vi "fgv_DL950_visa.vi"(7 "cmd":T2, 8 "error in":errorcluster, 10 "ms":u32, 11 "Initiate":string=":STAR;") -> (0 "error out":errorcluster, 2 "items":dbl[][](array[numeric]), 3 "Data":string)   [LabVIEW 2019]
uses:
  _ctrl/fgv_DL950.ctl
  _ctrl/init-r-stop.ctl
  _ctrl/rw.ctl
  SubVIs/common/cmd_err.ctl
  Durability/DL950_wfms.ctl
  d5429c9e-11ee-4f4d-90f7-2d4e6cc73670.vi
  SubVIs/common/Glob_Ref.vi
  Durability/common/Global 1.vi
  <instrlib>/Yokogawa DL950 Series/Public/Configure/Configure Module (Voltage).vi
  <instrlib>/Yokogawa DL950 Series/Public/Configure/Configure Module (Temperature).vi
  <instrlib>/Yokogawa DL950 Series/Yokogawa DL950 Series.lvlib
panel:
  out "resulting string":string
  out "Array":T1(array[cluster])
  in  "High":dbl
  in  "Middle":dbl
  in  "low":dbl
  in  "ch":i32
  out "DL950 wfm":waveform(dbl)[](graph)
  out "wf,":waveform(dbl)[](graph)
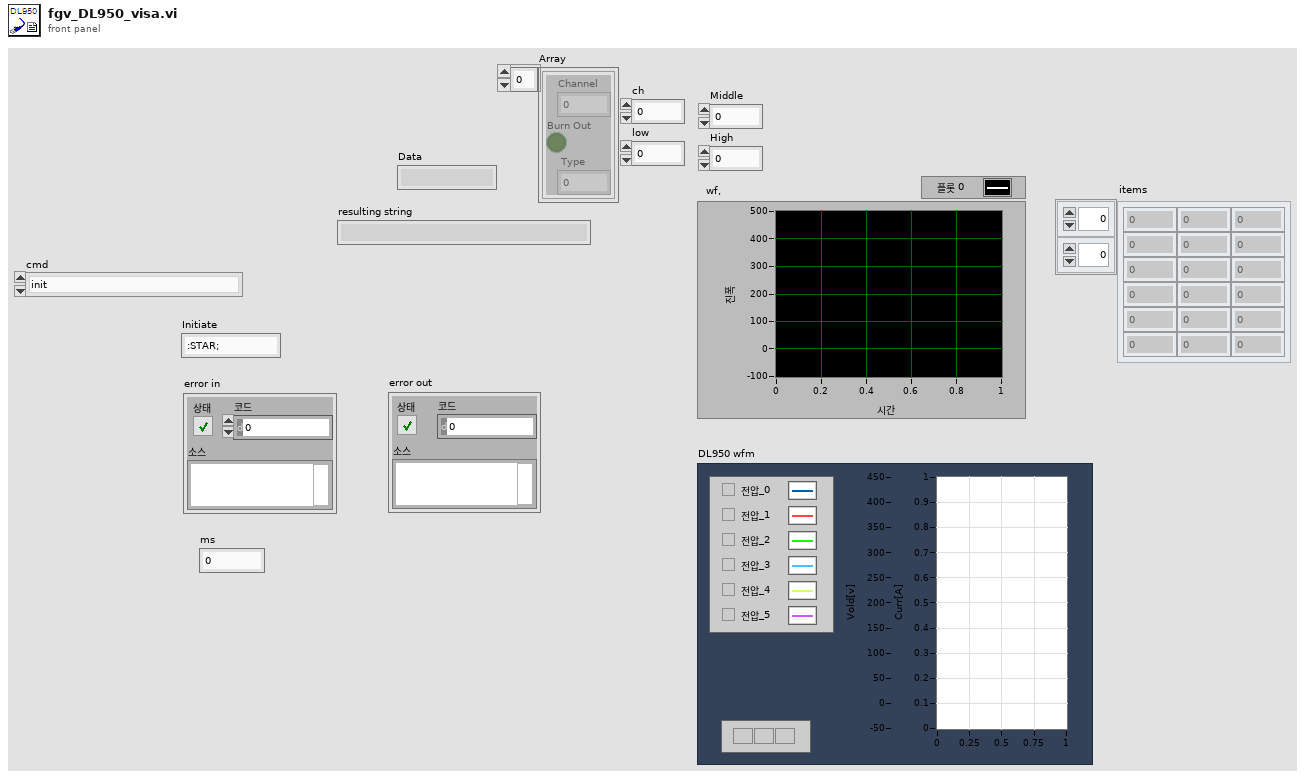
[diagram p1: front panel]
types:
  T1 = cluster{"Channel":u16, "Burn Out":bool, " Type ":i32}[]
  T2 = typedef "fgv_DL950.ctl" = enum16{"init", "config", "Set-NCh", "setapply", "trigger", "history_clear", "read", "time-div", "wave-aquis", "start", "query", "abort", "set_items", "reset_items", "read_items", "percent_rise", "trigger_single", "stop", "offset cancel", "close"}
  T3 = enum16{"DL950", "BP4610", "DSP1500", "cDAQ-AI", "cDAQ-AO", "cDAQ-DO"}
  T4 = typedef "init-r-stop.ctl" = enum16{"ini", "read", "stop"}
  T5 = typedef "cmd_err.ctl" = enum16{"close", "open", "default"}
  T6 = typedef "rw.ctl" = enum16{"read", "write"}
  T7 = typedef "DL950_wfms.ctl" = cluster{"wfms":waveform(dbl)[], "Waveform_2":cluster{"t0":dbl, "dt":dbl, "Y":dbl[][]}, "items":dbl[][], "da950_array":dbl[]}
  T8 = cluster{"Waveform_DLM5038":cluster{"l":dbl, "dt":dbl, "Y":dbl[][]}, "wf,":waveform(dbl)[]}
  T9 = typedef "DL950_config.ctl" = cluster{"Timeout":u32, "Time Div":i32, "Acq Mode":i32, "Record Len":i32, "Record Num":i32, "Start Point":i64, "End Poin":i64, "Visa":refnum<visa-resource-name>, "Config Voltage":cluster{"Enable":bool, "Ch":u16, "V Div":i32, "Coupling":i32, "Probe":i32, "Act.Items":bool, "items":i32[]}[], "Trigger on":bool, "Trigger Level":dbl, "Reset":bool, "Config Temp":cluster{"Channel":u16, "Burn Out":bool, " Type ":i32}[], "Trig Mode":i32, "Trig Pos":dbl, "Trigger Slope":i32, "Trigger Source ":i32, "Trig Start -5":dbl, "End 5":dbl}
  T10 = cluster{"Enable":bool, "Ch":u16, "V Div":i32, "Coupling":i32, "Probe":i32, "Act.Items":bool, "items":i32[]}[]
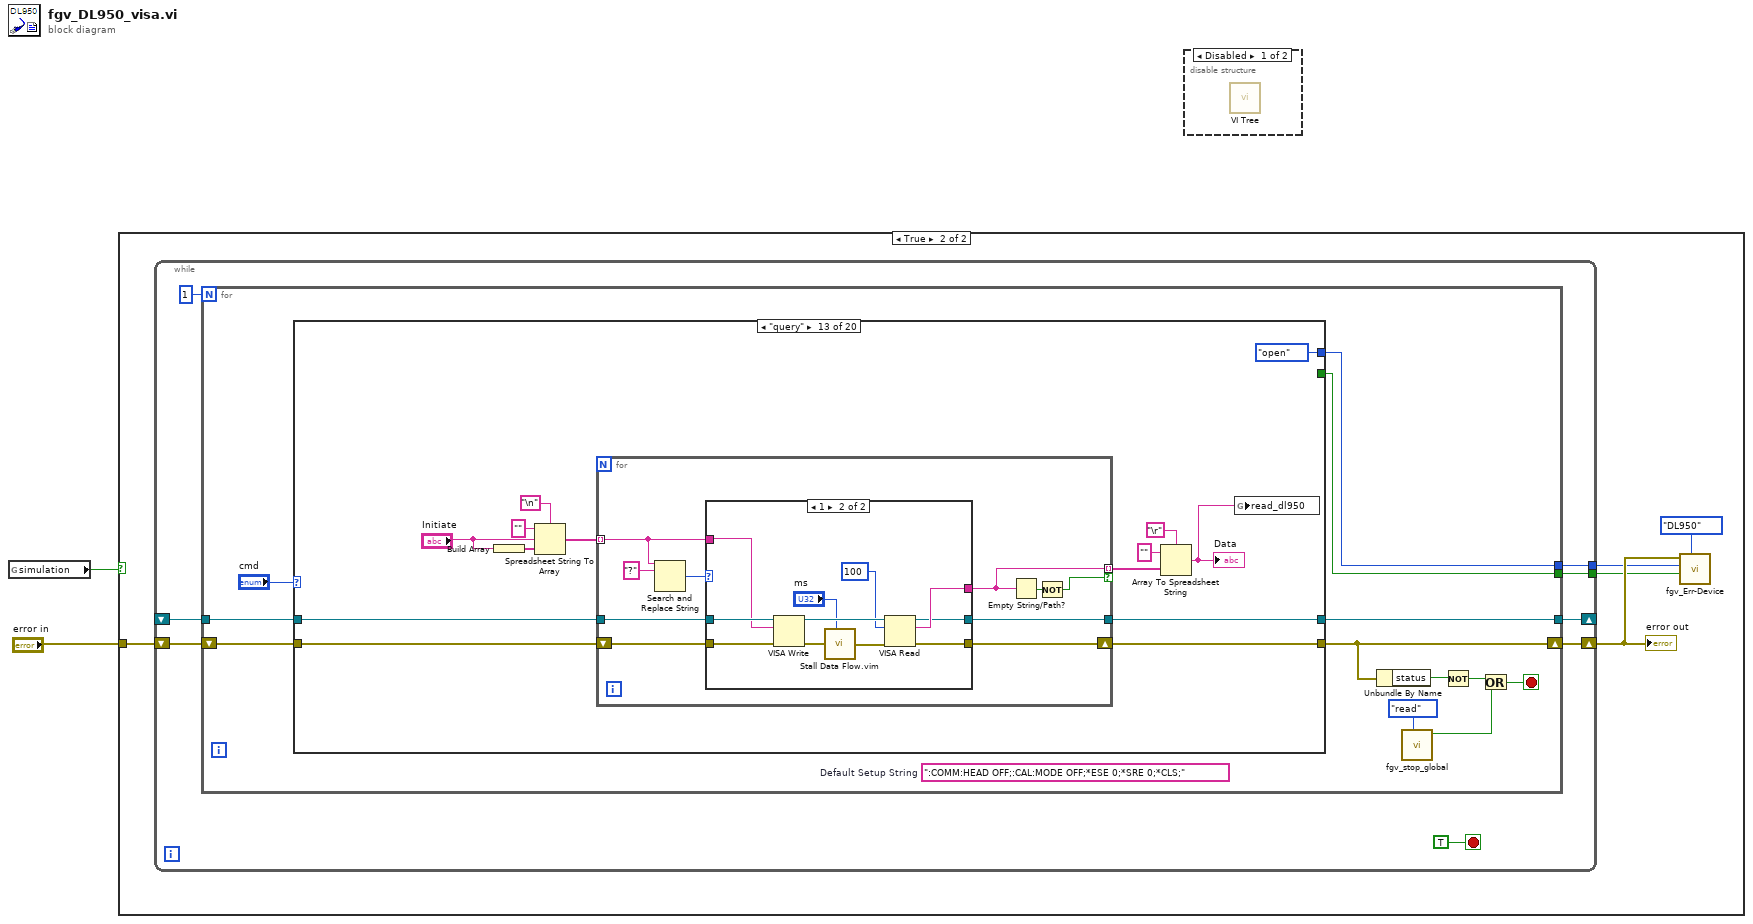
[diagram p0: block diagram]
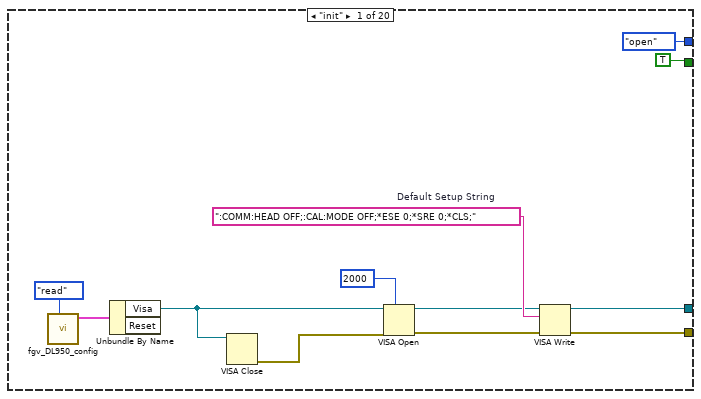
[diagram p3: hidden frame]
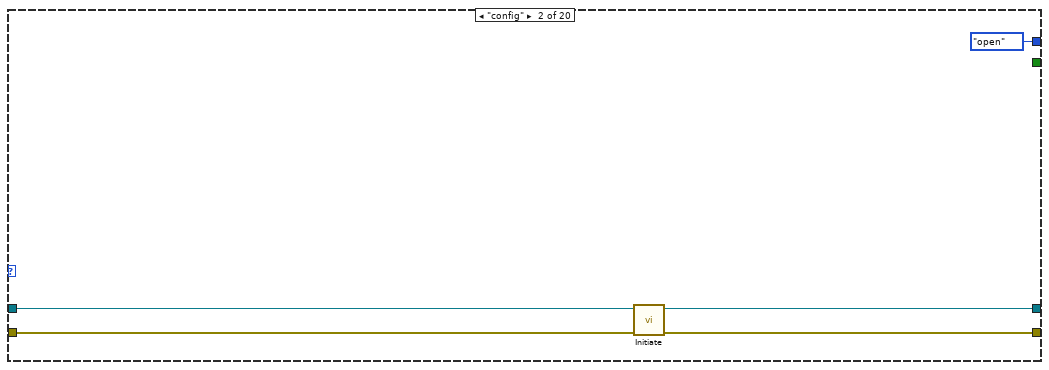
[diagram p4: hidden frame]
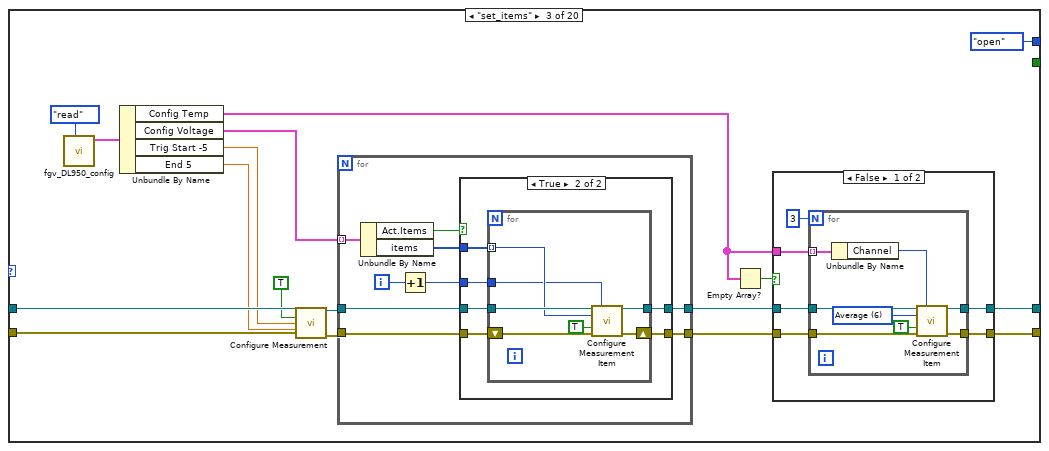
[diagram p5: hidden frame]
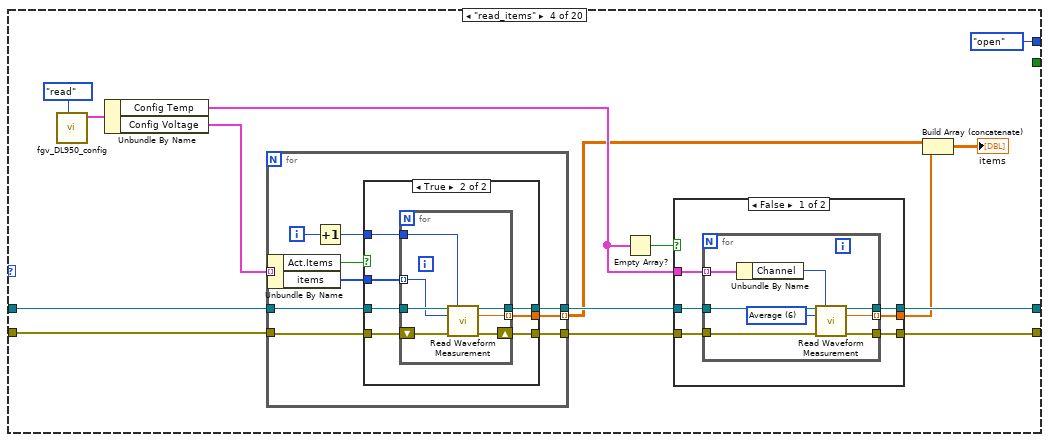
[diagram p8: hidden frame]
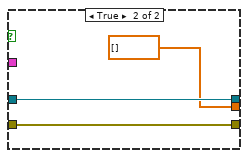
[diagram p9: hidden frame]
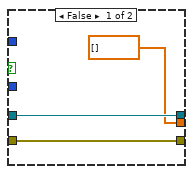
[diagram p10: hidden frame]
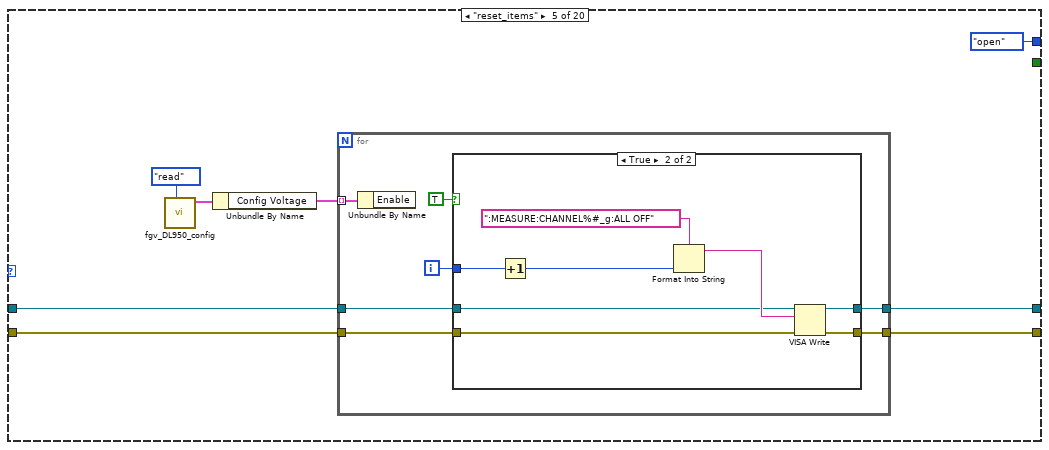
[diagram p11: hidden frame]
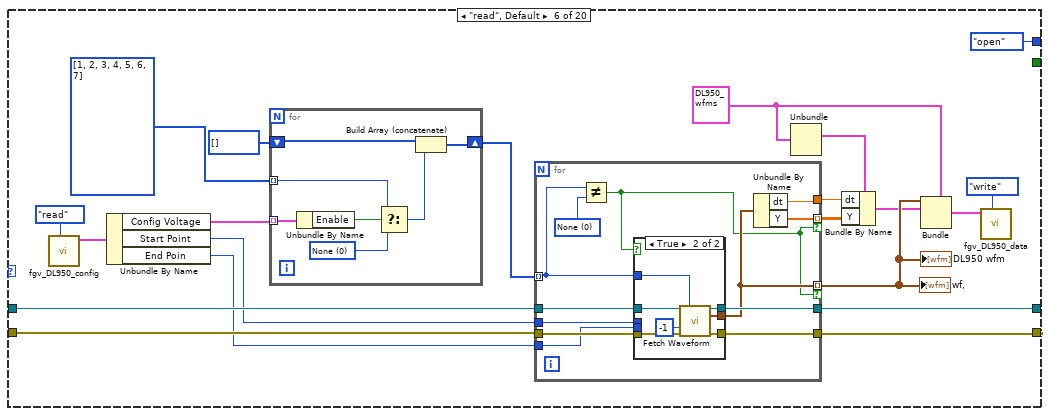
[diagram p13: hidden frame]
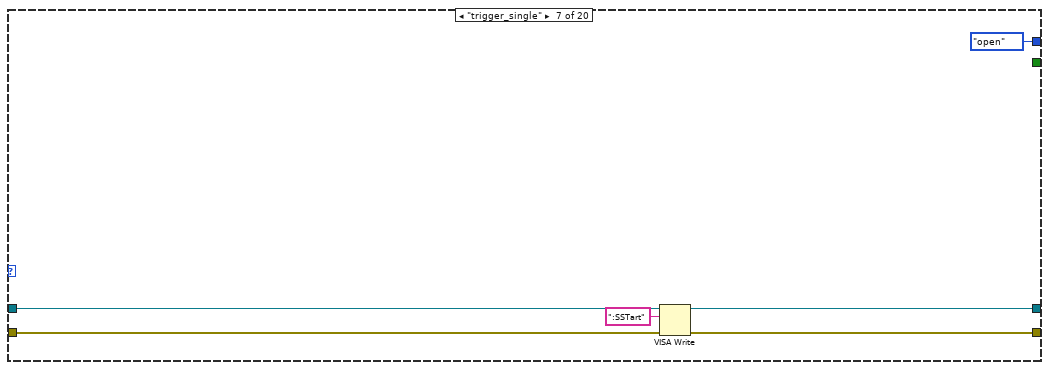
[diagram p15: hidden frame]
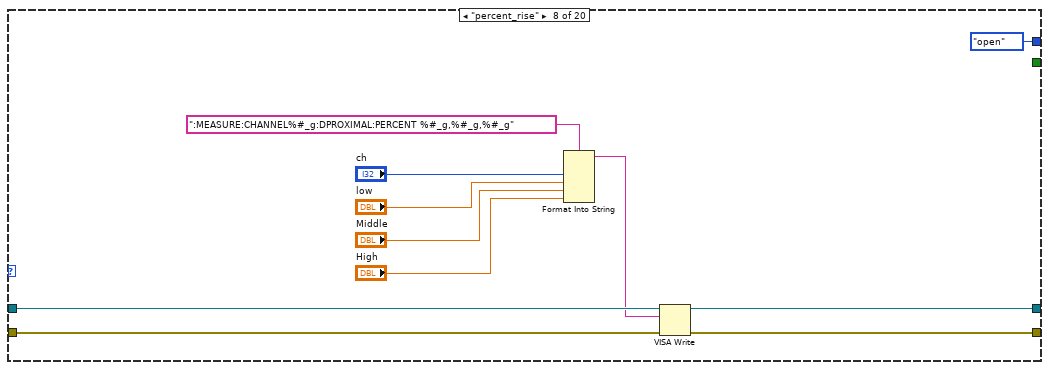
[diagram p16: hidden frame]
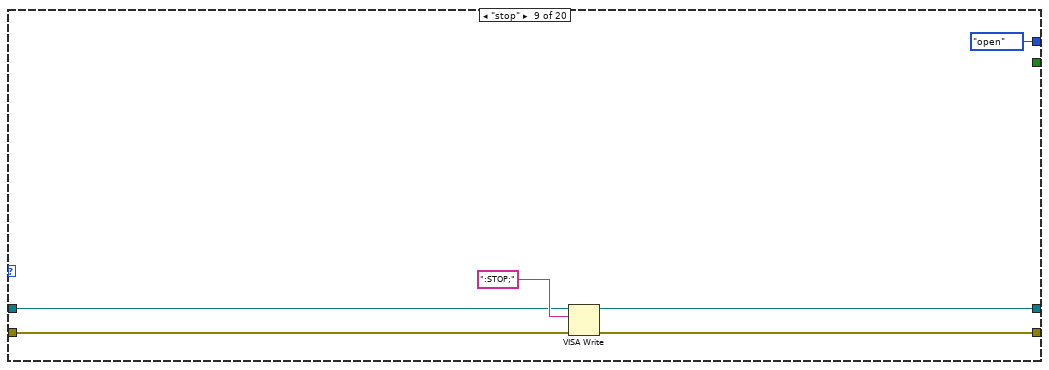
[diagram p17: hidden frame]
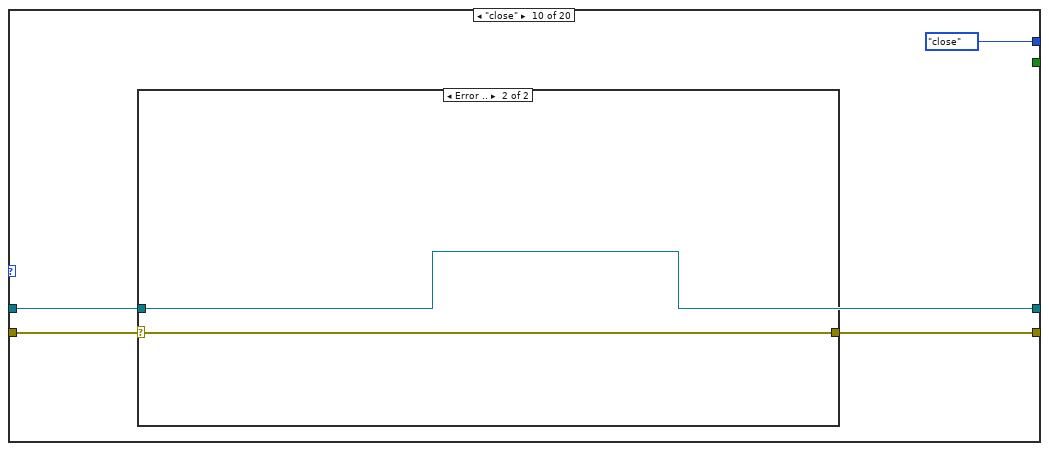
[diagram p18: hidden frame]
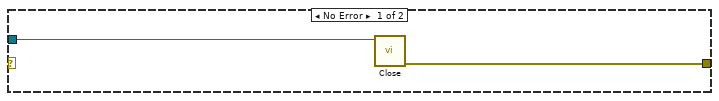
[diagram p19: hidden frame]
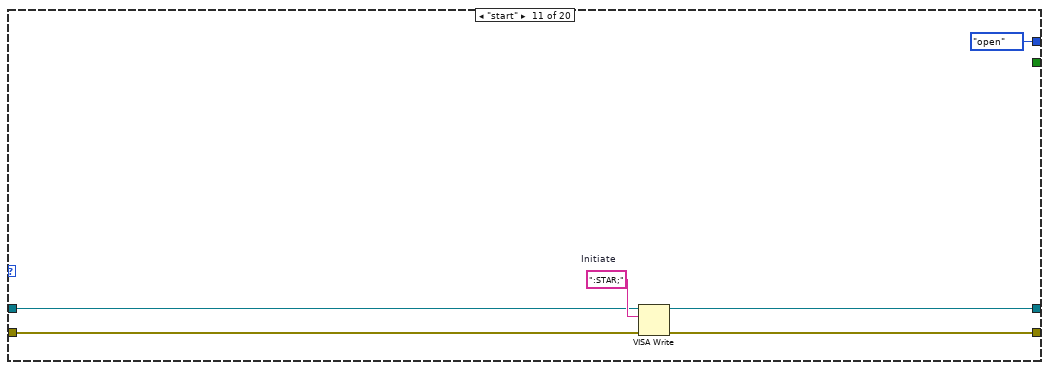
[diagram p20: hidden frame]
diagram:
  n1 = global read "Glob_Ref.vi" "simulation"() -> (w1:bool)
  n2 = case shown="True" w1 {
    tunnel: "error in" -> [_ w3]
    frame False {
    }
    frame True {
      n3 = while {
        shift-right: [w11] -> _
        shift-left: _ -> [w14]
        shift-right: [w12] -> w6
        shift-left: w3 -> [w13]
        tunnel: [w9] -> w5
        tunnel: [w8] -> w4
        stop <- TRUE stop-if-true
        n4 = for {
          N: 1 -> [_]
          tunnel: w14 -> [w26]
          tunnel: [w17] -> w11
          shift-right: [w16] -> w12
          shift-left: w13 -> [w25]
          tunnel: [w19] -> w9
          tunnel: [w18] -> w8
          stop <- w21 stop-if-true
          (unwired) ":COMM:HEAD OFF;:CAL:MODE OFF;*ESE 0;*SRE 0;*CLS;"  # Default Setup String
          n5 = case shown="\"query\"" "cmd" {
            tunnel: [w39 w44 w53 w106 w162 w196 w237 w248 w254 w260 w266 w275 w282 w322 w334 w382 w391 w433 w438 w488] -> w16
            tunnel: [w38 w43 w54 w107 w164 w198 w239 w250 w255 w261 w267 w276 w281 w321 w333 w383 w390 w432 w439 w489] -> w17
            tunnel: w26 -> [_ w42 w52 w114 w165 w199 w240 w251 w256 w261 w269 w278 w285 w320 w332 w385 w395 w431 w445 w493]
            tunnel: w25 -> [_ w41 w50 w113 w163 w197 w238 w249 w253 w258 w268 w277 w283 w323 w335 w384 w394 w434 w446 w494]
            tunnel: [cmd_err."open" ("cmd") cmd_err."open" ("cmd") cmd_err."open" ("cmd") cmd_err."open" ("cmd") cmd_err."open" ("cmd") cmd_err."open" ("cmd") cmd_err."open" ("cmd") cmd_err."open" ("cmd") cmd_err."open" ("cmd") cmd_err."close" ("cmd") cmd_err."open" ("cmd") cmd_err."open" ("cmd") cmd_err."open" ("cmd") cmd_err."open" ("cmd") cmd_err."open" ("cmd") _ cmd_err."open" ("cmd") cmd_err."open" ("cmd") cmd_err."open" ("cmd") cmd_err."open" ("cmd")] -> w19
            tunnel: [TRUE ("first?") _ _ _ _ _ _ _ _ _ _ _ _ _ _ _ _ _ _ _] -> w18
            frame "init" {
              w31 = ":COMM:HEAD OFF;:CAL:MODE OFF;*ESE 0;*SRE 0;*CLS;"  # Default Setup String
              n6 = call "fgv_DL950_config.vi"("cmd"=rw."read") -> ("config 2"=w36:T9)  [unwired: 9 in, 1 out]
              n7 = Unbundle By Name(w36) -> ("Visa"=w34:refnum<visa-resource-name>)  [unwired: 1 out]
              n8 = VISA Close ("VISAクローズ")(VISA resource name=w34) -> (error out=w33:errorcluster)  [unwired: 1 in]
              n9 = VISA Open ("VISAオープン")(timeout (0)=u32 2000 ("VISA Open timeout (0)"), error in (no error)=w33, VISA resource name=w34) -> (VISA resource name=w30:refnum<visa-resource-name>, error out=w29:errorcluster)  [unwired: 2 in]
              n10 = VISA Write ("VISA書き込み")(VISA resource name=w30, write buffer=w31, error in (no error)=w29) -> (VISA resource name out=w38:refnum<visa-resource-name>, error out=w39:errorcluster)  [unwired: 1 out]
            }
            frame "config" {
              n11 = call <instrlib>:"Initiate.vi"("error in (no error)"=w41, "VISA resource name"=w42) -> ("error out"=w44:errorcluster, "VISA resource name out"=w43:refnum<visa-resource-name>)  [unwired: 8 in]
            }
            frame "set_items" {
              n12 = call "fgv_DL950_config.vi"("cmd"=rw."read") -> ("config 2"=w60:T9)  [unwired: 9 in, 1 out]
              n13 = Unbundle By Name(w60) -> ("Config Temp"=w58:T1, "Config Voltage"=w59:T10, "Trig Start -5"=w48:dbl, "End 5"=w47:dbl)
              n14 = call <instrlib>:"Configure Measurement.vi"("VISA resource name"=w52, "Enable Measurement (True)"=TRUE, "Start Point (-5.00)"=w48, "End Point (5.00)"=w47, "error in (no error)"=w50) -> ("VISA resource name out"=w51:refnum<visa-resource-name>, "error out"=w49:errorcluster)  [unwired: 9 in]
              n15 = for {
                tunnel: w49 -> [w86]
                tunnel: [w85] -> w55
                tunnel: w51 -> [w84]
                tunnel: [w83] -> w56
                tunnel: w59 -> [w82] mode=indexing
                i -> [w79]
                n16 = Unbundle By Name(w82) -> ("Act.Items"=w81:bool, "items"=w80:i32[])
                n17 = Increment(x=w79) -> (x+1=w78:i32)
                n18 = case shown="True" w81 {
                  tunnel: w86 -> [w87 w94]
                  tunnel: [w87 w93] -> w85
                  tunnel: w84 -> [w88 w92]
                  tunnel: [w88 w91] -> w83
                  tunnel: w80 -> [_ w90]
                  tunnel: w78 -> [_ w89]
                  frame False {
                  }
                  frame True {
                    n19 = for {
                      tunnel: w92 -> [w99]
                      tunnel: [w98] -> w91
                      shift-right: [w100] -> w93
                      shift-left: w94 -> [w101]
                      tunnel: w90 -> [w96] mode=indexing
                      tunnel: w89 -> [w95]
                      n20 = call <instrlib>:"Configure Measurement Item.vi"("VISA resource name"=w99, "Source (1: CH1)"=w95, "Measurement Item (0: Peak to Peak)"=w96, "Enable Measurement Item (False)"=TRUE, "error in (no error)"=w101) -> ("VISA resource name out"=w98:refnum<visa-resource-name>, "error out"=w100:errorcluster)  [unwired: 9 in]
                    }
                  }
                }
              }
              n21 = Empty Array?(array=w58) -> (empty?=w57:bool)
              n22 = case shown="False" w57 {
                tunnel: w58 -> [w67 _]
                tunnel: w56 -> [w66 w77]
                tunnel: w55 -> [w65 w76]
                tunnel: [w64 w77] -> w54
                tunnel: [w63 w76] -> w53
                frame False {
                  n23 = for {
                    N: 3 -> [_]
                    tunnel: w67 -> [w72] mode=indexing
                    tunnel: w66 -> [w74]
                    tunnel: w65 -> [w73]
                    tunnel: [w69] -> w64
                    tunnel: [w68] -> w63
                    w70 = 6 items=["Peak to Peak", "Amplitude", "Max", "Min", "High", "Low", "Average", "Middle", "Rms", "Standard Deviation", "+Overshoot", "-Overshoot", "Rise", "Fall", "Frequency", "Period", "+Width", "-Width", "Duty Cycle", "Pulse Count", "Burst1 Width", "Burst2 Width", "Average Frequency", "Average Period", "Int1TY", "Int2TY"] ("Measurement Item (0: Peak to Peak)")
                    n24 = Unbundle By Name(w72) -> ("Channel"=w71:u16)
                    n25 = call <instrlib>:"Configure Measurement Item.vi"("VISA resource name"=w74, "Source (1: CH1)"=w71, "Measurement Item (0: Peak to Peak)"=w70, "Enable Measurement Item (False)"=TRUE, "error in (no error)"=w73) -> ("VISA resource name out"=w69:refnum<visa-resource-name>, "error out"=w68:errorcluster)  [unwired: 9 in]
                  }
                }
                frame True {
                }
              }
            }
            frame "read_items" {
              n26 = call "fgv_DL950_config.vi"("cmd"=rw."read") -> ("config 2"=w115:T9)  [unwired: 9 in, 1 out]
              n27 = Unbundle By Name(w115) -> ("Config Temp"=w109:T1, "Config Voltage"=w112:T10)
              n28 = for {
                tunnel: w113 -> [w143]
                tunnel: [w142] -> w110
                tunnel: w114 -> [w141]
                tunnel: [w140] -> w111
                tunnel: w112 -> [w139] mode=indexing
                tunnel: [w134] -> w105 mode=indexing
                i -> [w136]
                n29 = Unbundle By Name(w139) -> ("Act.Items"=w138:bool, "items"=w137:i32[])
                n30 = Increment(x=w136) -> (x+1=w135:i32)
                n31 = case shown="True" w138 {
                  tunnel: w143 -> [w145 w153]
                  tunnel: [w145 w152] -> w142
                  tunnel: w141 -> [w146 w151]
                  tunnel: [w146 w150] -> w140
                  tunnel: w137 -> [_ w149]
                  tunnel: w135 -> [_ w148]
                  tunnel: [dbl[] [] w147] -> w134
                  frame False {
                  }
                  frame True {
                    n32 = for {
                      tunnel: w151 -> [w160]
                      tunnel: [w158] -> w150
                      shift-right: [w157] -> w152
                      shift-left: w153 -> [w159]
                      tunnel: w149 -> [w156] mode=indexing
                      tunnel: w148 -> [w155]
                      tunnel: [w154] -> w147 mode=indexing
                      n33 = call <instrlib>:"Read Waveform Measurement.vi"("VISA resource name"=w160, "Source (1: CH1)"=w155, "Measurement Item (0: Peak to Peak)"=w156, "error in (no error)"=w159) -> ("VISA resource name out"=w158:refnum<visa-resource-name>, "Measurement Value"=w154:dbl, "error out"=w157:errorcluster)  [unwired: 9 in]
                    }
                  }
                }
              }
              n34 = Empty Array?(array=w109) -> (empty?=w108:bool)
              n35 = case shown="False" w108 {
                tunnel: w111 -> [w122 w133]
                tunnel: w110 -> [w121 w132]
                tunnel: w109 -> [w120 _]
                tunnel: [w119 w133] -> w107
                tunnel: [w118 w132] -> w106
                tunnel: [w117 dbl[] []] -> w104
                frame False {
                  n36 = for {
                    tunnel: w121 -> [w130]
                    tunnel: [w129] -> w118
                    tunnel: w122 -> [w128]
                    tunnel: [w127] -> w119
                    tunnel: w120 -> [w126] mode=indexing
                    tunnel: [w125] -> w117 mode=indexing
                    w124 = 6 items=["Peak to Peak", "Amplitude", "Max", "Min", "High", "Low", "Average", "Middle", "Rms", "Standard Deviation", "+Overshoot", "-Overshoot", "Rise", "Fall", "Frequency", "Period", "+Width", "-Width", "Duty Cycle", "Pulse Count", "Burst1 Width", "Burst2 Width", "Average Frequency", "Average Period", "Int1TY", "Int2TY", "Delay"] ("Measurement Item (0: Peak to Peak)")
                    n37 = Unbundle By Name(w126) -> ("Channel"=w123:u16)
                    n38 = call <instrlib>:"Read Waveform Measurement.vi"("VISA resource name"=w128, "Source (1: CH1)"=w123, "Measurement Item (0: Peak to Peak)"=w124, "error in (no error)"=w130) -> ("VISA resource name out"=w127:refnum<visa-resource-name>, "Measurement Value"=w125:dbl, "error out"=w129:errorcluster)  [unwired: 9 in]
                  }
                }
                frame True {
                }
              }
              n39 = Build Array (concatenate)(w105, w104) -> (→"items":dbl[][])
            }
            frame "reset_items" {
              n40 = call "fgv_DL950_config.vi"("cmd"=rw."read") -> ("config 2"=w167:T9)  [unwired: 9 in, 1 out]
              n41 = Unbundle By Name(w167) -> ("Config Voltage"=w166:T10)
              n42 = for {
                tunnel: w166 -> [w175] mode=indexing
                tunnel: w165 -> [w173]
                tunnel: [w172] -> w164
                tunnel: w163 -> [w171]
                tunnel: [w170] -> w162
                i -> [w174]
                n43 = Unbundle By Name(w175) -> ()  [unwired: 1 out]
                n44 = case shown="True" TRUE {
                  tunnel: w174 -> [_ w184]
                  tunnel: w173 -> [w177 w181]
                  tunnel: [w177 w180] -> w172
                  tunnel: w171 -> [w176 w179]
                  tunnel: [w176 w178] -> w170
                  frame False {
                  }
                  frame True {
                    n45 = Increment(x=w184) -> (x+1=w183:i32)
                    n46 = Format Into String(format string=":MEASURE:CHANNEL%#_g:ALL OFF", w183) -> (resulting string=w182:string)  [unwired: 2 in, 1 out]
                    n47 = VISA Write(VISA resource name=w181, write buffer=w182, error in (no error)=w179) -> (VISA resource name out=w180:refnum<visa-resource-name>, error out=w178:errorcluster)  [unwired: 1 out]
                  }
                }
              }
            }
            frame "read", Default {
              w189 = T7 {"wfms"=[], "Waveform_2"={"t0"=0.0, "dt"=0.0, "Y"=[]}, "items"=[], "da950_array"=[10.0, 0.02, 0.074492, 0.033331, 0.018948904, 3.5928321, 0.0, 0.0, 400.375, 399.625, 3.5928321, 0.0, 0.0, 0.074492, 0.0, 0.0]} ("DL950 wfm")
              w201 = u16[] [1, 2, 3, 4, 5, 6, 7] items=["None", "CH1", "CH2", "CH3", "CH4", "CH5", "CH6", "CH7", "CH8", "CH9", "CH10", "CH11", "CH12", "CH13", "CH14", "CH15", "CH16", "MATH1", "MATH2", "MATH3", "MATH4", "MATH5", "MATH6", "MATH7", "MATH8", "EVENT"] ("Source (1: CH1)")
              n48 = call "fgv_DL950_config.vi"("cmd"=rw."read") -> ("config 2"=w204:T9)  [unwired: 9 in, 1 out]
              n49 = Unbundle By Name(w204) -> ("Config Voltage"=w203:T10, "Start Point"=w195:i64, "End Poin"=w194:i64)
              n50 = for {
                tunnel: w203 -> [w234] mode=indexing
                shift-right: [w232] -> w200
                shift-left: u16[] [] -> [w233]
                tunnel: w201 -> [w230] mode=indexing
                w229 = u16 0 items=["None", "CH1", "CH2", "CH3", "CH4", "CH5", "CH6", "CH7", "CH8", "CH9", "CH10", "CH11", "CH12", "CH13", "CH14", "CH15", "CH16", "MATH1", "MATH2", "MATH3", "MATH4", "MATH5", "MATH6", "MATH7", "MATH8", "EVENT"]
                n51 = Unbundle By Name(w234) -> ("Enable"=w231:bool)
                n52 = Select(t=w230, s=w231, f=w229) -> (s? t:f=w228:u16)
                n53 = Build Array (concatenate)(w233, w228) -> (w232:u16[])
              }
              n54 = for {
                tunnel: w200 -> [w209] mode=indexing
                tunnel: w199 -> [w218]
                tunnel: [w217] -> w198
                tunnel: w197 -> [w216]
                tunnel: [w215] -> w196
                tunnel: w195 -> [w214]
                tunnel: w194 -> [w213]
                tunnel: [w212] -> w193
                tunnel: [w211] -> w192 mode=indexing if=w207
                tunnel: [w210] -> w190 mode=indexing if=w207
                w208 = u16 0 items=["None", "CH1", "CH2", "CH3", "CH4", "CH5", "CH6", "CH7", "CH8", "CH9", "CH10", "CH11", "CH12", "CH13", "CH14", "CH15", "CH16", "MATH1", "MATH2", "MATH3", "MATH4", "MATH5", "MATH6", "MATH7", "MATH8", "EVENT"] ("Ch")
                n55 = Not Equal?(x=w209, y=w208) -> (x != y?=w207:bool)
                n56 = case shown="True" w207 {
                  tunnel: w218 -> [w220 w227]
                  tunnel: [w220 w226] -> w217
                  tunnel: w216 -> [w219 w225]
                  tunnel: [w219 w224] -> w215
                  tunnel: w214 -> [_ _]
                  tunnel: w213 -> [_ _]
                  tunnel: [_ w223] -> w210
                  tunnel: w209 -> [_ w222]
                  frame False {
                  }
                  frame True {
                    n57 = call <instrlib>:"Fetch Waveform.vi"("VISA resource name"=w227, "Source (1: CH1)"=w222, "End Point(1000)"=i64 -1, "error in (no error)"=w225) -> ("VISA resource name out"=w226:refnum<visa-resource-name>, "Waveform Data"=w223:waveform(dbl), "error out"=w224:errorcluster)  [unwired: 9 in]
                  }
                }
                n58 = Unbundle By Name(w210) -> ("dt"=w212:dbl, "Y"=w211:dbl[])
              }
              "wf," <- w190
              "DL950 wfm" <- w190
              n59 = Unbundle(w189) -> ("Waveform_2"=w188:cluster{"t0":dbl, "dt":dbl, "Y":dbl[][]})  [unwired: 3 out]
              n60 = Bundle By Name(cluster=w188, "dt"=w193, "Y"=w192) -> (w187:cluster{"t0":dbl, "dt":dbl, "Y":dbl[][]})
              n61 = Bundle(cluster=w189, "wfms"=w190, "Waveform_2"=w187) -> (w191:T7)  [unwired: 2 in]
              n62 = call "fgv_DL950_data.vi"("cmd"=rw."write", "DL950 wfm"=w191) -> ()  [unwired: 8 in, 2 out]
            }
            frame "trigger_single" {
              n63 = VISA Write(VISA resource name=w240, write buffer=":SSTart", error in (no error)=w238) -> (VISA resource name out=w239:refnum<visa-resource-name>, error out=w237:errorcluster)  [unwired: 1 out]
            }
            frame "percent_rise" {
              n64 = Format Into String(format string=":MEASURE:CHANNEL%#_g:DPROXIMAL:PERCENT %#_g,%#_g,%#_g", "ch", "low", "Middle", "High") -> (resulting string=w242:string)  [unwired: 2 in, 1 out]
              n65 = VISA Write(VISA resource name=w251, write buffer=w242, error in (no error)=w249) -> (VISA resource name out=w250:refnum<visa-resource-name>, error out=w248:errorcluster)  [unwired: 1 out]
            }
            frame "stop" {
              n66 = VISA Write ("VISA書き込み")(VISA resource name=w256, write buffer=":STOP;", error in (no error)=w253) -> (VISA resource name out=w255:refnum<visa-resource-name>, error out=w254:errorcluster)  [unwired: 1 out]
            }
            frame "close" {
              n67 = case shown="Error .." w258 {
                selector: w258 -> [_ w264]
                tunnel: w261 -> [w263 _]
                tunnel: [w262 w264] -> w260
                frame No Error {
                  n68 = call <instrlib>:"Close.vi"("VISA resource name"=w263) -> ("error out"=w262:errorcluster)  [unwired: 10 in]
                }
                frame Error {
                }
              }
            }
            frame "start" {
              w270 = ":STAR;"  # Initiate
              n69 = VISA Write ("VISA書き込み")(VISA resource name=w269, write buffer=w270, error in (no error)=w268) -> (VISA resource name out=w267:refnum<visa-resource-name>, error out=w266:errorcluster)  [unwired: 1 out]
            }
            frame "offset cancel" {
              w271 = 6.0  # ch
              w273 = ":CHANNEL%#_g:VOLTAGE:DOCANCEL:EXECUTE;"  # Initiate
              n70 = Format Into String(format string=w273, w271) -> (resulting string=w272:string)  [unwired: 2 in, 1 out]
              "resulting string" <- w272
              n71 = VISA Write ("VISA書き込み")(VISA resource name=w278, write buffer=w272, error in (no error)=w277) -> (VISA resource name out=w276:refnum<visa-resource-name>, error out=w275:errorcluster)  [unwired: 1 out]
            }
            frame "query" {
              n72 = Build Array("Initiate") -> (w291:string[])
              n73 = Spreadsheet String To Array(delimiter (Tab)="\n", format string="", spreadsheet string="Initiate", array type (2D Dbl)=w291) -> (array=w284:string[])
              n74 = for {
                tunnel: w285 -> [w295]
                shift-right: [w300] -> w282
                shift-left: w283 -> [w297]
                tunnel: w284 -> [w296] mode=indexing
                tunnel: [w294] -> w292 mode=indexing if=w299
                tunnel: [w293] -> w281
                n75 = Search and Replace String(input string=w296, search string="?" ("õ¶ñ")) -> (number of replacements=w301:i32)  [unwired: 6 in, 3 out]
                n76 = case shown="1" w301 {
                  tunnel: [w304 w314] -> w300
                  tunnel: w297 -> [w307 w308]
                  tunnel: w296 -> [w306 w313]
                  tunnel: w295 -> [w305 w316]
                  tunnel: [_ w315] -> w294
                  tunnel: [w303 w312] -> w293
                  frame 0, Default {
                    n77 = VISA Write(VISA resource name=w305, write buffer=w306, error in (no error)=w307) -> (VISA resource name out=w303:refnum<visa-resource-name>, error out=w304:errorcluster)  [unwired: 1 out]
                  }
                  frame 1 {
                    n78 = VISA Write(VISA resource name=w316, write buffer=w313, error in (no error)=w308) -> (VISA resource name out=w318:refnum<visa-resource-name>, error out=w311:errorcluster)  [unwired: 1 out]
                    n79 = call "Stall Data Flow.vim"("value in"=w311, "milliseconds to wait"="ms") -> ("value out"=w310:errorcluster)  [unwired: 1 out]
                    n80 = VISA Read(VISA resource name=w318, byte count=u32 100, error in (no error)=w310) -> (VISA resource name out=w312:refnum<visa-resource-name>, read buffer=w315:string, error out=w314:errorcluster)  [unwired: 1 out]
                  }
                }
                n81 = Empty String/Path?(string/path=w294) -> (empty?=w298:bool)
                n82 = Not(x=w298) -> (.not. x?=w299:bool)
              }
              n83 = Array To Spreadsheet String(delimiter (Tab)="\r", array=w292, 3:"" ("format string")) -> (spreadsheet string=w280:string)
              "Data" <- w280
              n84 = global write "Global 1.vi" "read_dl950"(w280) -> ()
            }
            frame "abort" {
              n85 = call <instrlib>:"Abort.vi"("error in (no error)"=w323, "VISA resource name"=w320) -> ("error out"=w322:errorcluster, "VISA resource name out"=w321:refnum<visa-resource-name>)  [unwired: 8 in]
            }
            frame "wave-aquis" {
              n86 = call "fgv_DL950_config.vi"("cmd"=rw."read") -> ("config 2"=w330:T9)  [unwired: 9 in, 1 out]
              n87 = Unbundle By Name(w330) -> ("Config Voltage"=w326:T10, "Record Num"=w329:i32, "Start Point"=w328:i64, "End Poin"=w327:i64)
              n88 = case shown="True" TRUE {
                tunnel: w335 -> [w337 w356]
                tunnel: [w336 w355] -> w334
                tunnel: [w341 w354] -> w333
                tunnel: w332 -> [w340 w353]
                tunnel: w329 -> [w339 w352]
                tunnel: w328 -> [_ w351]
                tunnel: w327 -> [w338 w350]
                tunnel: [w342 w349] -> _
                tunnel: w326 -> [_ w348]
                frame False {
                  n89 = call "waveAquis.vi"("End Point(1000)"=w338, "error in (no error)"=w337, "Record Number (0)"=w339, "VISA resource name"=w340) -> ("error out"=w336:errorcluster, "Waveform Data"=w342:waveform(dbl), "VISA resource name out"=w341:refnum<visa-resource-name>)  [unwired: 5 in]
                }
                frame True {
                  n90 = for {
                    tunnel: w356 -> [w369]
                    tunnel: [w368] -> w355
                    tunnel: [w367] -> w354
                    tunnel: w353 -> [w366]
                    tunnel: w352 -> [w365]
                    tunnel: w351 -> [w364]
                    tunnel: w350 -> [w363]
                    tunnel: [w357] -> w349
                    tunnel: w348 -> [w362] mode=indexing
                    tunnel: [w359] -> w346
                    tunnel: [w358] -> w345 mode=indexing
                    tunnel: [w357] -> w343 mode=indexing
                    i -> [w360]
                    n91 = Unbundle By Name(w362) -> ("Enable"=w361:bool)
                    n92 = case shown="True" w361 {
                      tunnel: w369 -> [w370 w381]
                      tunnel: [w370 w380] -> w368
                      tunnel: [w371 w379] -> w367
                      tunnel: w366 -> [w371 w378]
                      tunnel: w365 -> [_ w377]
                      tunnel: w364 -> [_ w376]
                      tunnel: w363 -> [_ w375]
                      tunnel: [_ w374] -> w357
                      tunnel: w360 -> [_ w373]
                      frame False {
                      }
                      frame True {
                        n93 = Increment(x=w373) -> (x+1=w372:i32)
                        n94 = call "waveAquis.vi"("End Point(1000)"=w375, "Source (1: CH1)"=w372, "error in (no error)"=w381, "Start Point(0)"=w376, "Record Number (0)"=w377, "VISA resource name"=w378) -> ("error out"=w380:errorcluster, "Waveform Data"=w374:waveform(dbl), "VISA resource name out"=w379:refnum<visa-resource-name>)  [unwired: 3 in]
                      }
                    }
                    n95 = Unbundle By Name(w357) -> ("dt"=w359:dbl, "Y"=w358:dbl[])
                  }
                  n96 = Bundle By Name(cluster=T8 {"Waveform_DLM5038"={"l"=0.0, "dt"=0.0, "Y"=[]}, "wf,"=[]} ("Waveform_DLM5038"), "Waveform_DLM5038.dt"=w346, "Waveform_DLM5038.Y"=w345) -> ()  [unwired: 1 out]
                  n97 = Bundle(cluster=T7 {"wfms"=[], "Waveform_2"={"t0"=0.0, "dt"=0.0, "Y"=[]}, "items"=[], "da950_array"=[10.0, 0.02, 0.074492, 0.033331, 0.018948904, 3.5928321, 0.0, 0.0, 400.375, 399.625, 3.5928321, 0.0, 0.0, 0.074492, 0.0, 0.0]} ("DL950 wfm"), "wfms"=w343) -> ()  [unwired: 3 in, 1 out]
                }
              }
            }
            frame "history_clear" {
              n98 = VISA Write ("VISA書き込み")(VISA resource name=w385, write buffer=":HISTory:CLEar;", error in (no error)=w384) -> (VISA resource name out=w383:refnum<visa-resource-name>, error out=w382:errorcluster)  [unwired: 1 out]
            }
            frame "setapply" {
              n99 = call "fgv_DL950_config.vi"("cmd"=rw."read") -> ("config 2"=w398:T9)  [unwired: 9 in, 1 out]
              n100 = Unbundle By Name(w398) -> ("Config Voltage"=w392:T10, "Time Div"=w393:i32, "Record Len"=w397:i32, "Acq Mode"=w396:i32)
              n101 = call <instrlib>:"Configure Acquisition.vi"("VISA resource name"=w395, "Record Length (0: 10k)"=w397, "Acquisition Mode (0: Normal)"=w396, "error in (no error)"=w394) -> ("VISA resource name out"=w400:refnum<visa-resource-name>, "error out"=w401:errorcluster)  [unwired: 10 in]
              n102 = call <instrlib>:"Configure Timebase.vi"("VISA resource name"=w400, "Time Division (12: 1ms)"=w393, "error in (no error)"=w401) -> ("VISA resource name out"=w389:refnum<visa-resource-name>, "error out"=w388:errorcluster)  [unwired: 11 in]
              n103 = for {
                tunnel: w392 -> [w407] mode=indexing
                tunnel: [w409] -> w391
                tunnel: [w408] -> w390
                tunnel: w389 -> [w403]
                tunnel: w388 -> [w402]
                i -> [w410]
                n104 = Unbundle By Name(w407) -> ("Enable"=w406:bool, "Coupling"=w405:i32, "V Div"=w404:i32)
                n105 = case shown="True" w406 {
                  tunnel: w410 -> [_ w426]
                  tunnel: [w411 w419] -> w409
                  tunnel: [w412 w418] -> w408
                  tunnel: w405 -> [_ w416]
                  tunnel: w404 -> [_ w415]
                  tunnel: w403 -> [w412 w414]
                  tunnel: w402 -> [w411 w413]
                  frame False {
                  }
                  frame True {
                    n106 = Increment(x=w426) -> (x+1=w417:i32)
                    n107 = Format Into String ("文字列にフォーマット")(format string="CHAN%d:", w417) -> (resulting string=w424:string)  [unwired: 2 in, 1 out]
                    n108 = Pick Line ("ライン選択")(string ("")=w424, multi-line string="COUP AC;\nCOUP DC;\nCOUP GND;\nCOUP ACRMS;\nCOUP DCRMS;", line index=w416) -> (output string=w425:string)
                    n109 = Pick Line ("ライン選択")(string ("")=w425, multi-line string="VDIV 0.0001;\nVDIV 0.0002;\nVDIV 0.0005;\nVDIV 0.001;\nVDIV 0.002;\nVDIV 0.005;\nVDIV 0.01;\nVDIV 0.02;\nVDIV 0.05;\nVDIV 0.1;\nVDIV 0.2;\nVDIV 0.5;\nVDIV 1;\nVDIV 2;\nVDIV 4;\nVDIV 5;\nVDIV 8;\nVDIV 10;\nVDIV 20;\nVDIV 40;\nVDIV 50;\nVDIV 80;\nVDIV 100;\nVDIV 200;\nVDIV 400;\nVDIV 500;\nVDIV 800;\nVDIV 1000;\nVDIV 2000;\nVDIV 4000;\nVDIV 5000;\nVDIV 8000;\nVDIV 10000;\nVDIV 20000;\nVDIV 25000;\nVDIV 50000;\nVDIV 100000;\nVDIV 250000;\nVDIV 500000;\nVDIV 1000000;", line index=w415) -> (output string=w423:string)
                    n110 = VISA Write ("VISA書き込み")(VISA resource name=w414, write buffer=w423, error in (no error)=w413) -> (VISA resource name out=w418:refnum<visa-resource-name>, error out=w419:errorcluster)  [unwired: 1 out]
                  }
                }
              }
            }
            frame "time-div" {
              n111 = call "fgv_DL950_config.vi"("cmd"=rw."read") -> ("config 2"=w429:T9)  [unwired: 9 in, 1 out]
              n112 = Unbundle By Name(w429) -> ("Time Div"=w428:i32)
              n113 = call <instrlib>:"Configure Timebase.vi"("VISA resource name"=w431, "Time Division (12: 1ms)"=w428, "error in (no error)"=w434) -> ("VISA resource name out"=w432:refnum<visa-resource-name>, "error out"=w433:errorcluster)  [unwired: 11 in]
            }
            frame "Set-NCh" {
              n114 = call "fgv_DL950_config.vi"("cmd"=rw."read") -> ("config 2"=w443:T9)  [unwired: 9 in, 1 out]
              n115 = Unbundle By Name(w443) -> ("Config Temp"=w436:T1, "Config Voltage"=w442:T10)
              n116 = for {
                tunnel: w446 -> [w473]
                tunnel: [w472] -> w440
                tunnel: w445 -> [w471]
                tunnel: [w470] -> w441
                tunnel: w442 -> [w469] mode=indexing
                n117 = Unbundle By Name(w469) -> ("Enable"=w466:bool, "Ch"=w464:u16, "Coupling"=w465:i32, "Probe"=w468:i32, "V Div"=w467:i32)
                n118 = case shown="True" w466 {
                  tunnel: w473 -> [w474 w483]
                  tunnel: [w474 w482] -> w472
                  tunnel: w471 -> [w475 w481]
                  tunnel: [w475 w480] -> w470
                  tunnel: w465 -> [_ w479]
                  tunnel: w468 -> [_ w477]
                  tunnel: w467 -> [_ w478]
                  tunnel: w464 -> [_ w476]
                  frame False {
                  }
                  frame True {
                    n119 = call-poly <instrlib>:"Configure Module.vi"("VISA resource name"=w481, "Channel (1: CH1)"=w476, "Vertical Coupling (1: DC)"=w479, "Probe Attenuation (3: 10:1)"=w477, "Vertical Division (20: 50)"=w478, "error in (no error)"=w483) -> ("VISA resource name out"=w480:refnum<visa-resource-name>, "error out"=w482:errorcluster)  [unwired: 8 in]
                  }
                }
              }
              n120 = Empty Array?(array=w436) -> (empty?=w437:bool)
              n121 = case shown="False" w437 {
                tunnel: w441 -> [w453 w463]
                tunnel: w440 -> [w452 w462]
                tunnel: [w451 w463] -> w439
                tunnel: [w450 w462] -> w438
                tunnel: w436 -> [w449 _]
                frame False {
                  n122 = for {
                    N: 3 -> [_]
                    shift-right: [w459] -> w451
                    shift-left: w453 -> [w461]
                    shift-right: [w458] -> w450
                    shift-left: w452 -> [w460]
                    tunnel: w449 -> [w454] mode=indexing
                    tunnel: [w454] -> w447 mode=indexing
                    n123 = Unbundle By Name(w454) -> ("Channel"=w457:u16, "Burn Out"=w456:bool, "Type"=w455:i32)
                    n124 = call-poly <instrlib>:"Configure Module.vi"("VISA resource name"=w461, "Channel (1: CH1)"=w457, "Enable Burn Out (F:Off)"=w456, "Thermocouple Type (0: K)"=w455, "error in (no error)"=w460) -> ("VISA resource name out"=w459:refnum<visa-resource-name>, "error out"=w458:errorcluster)  [unwired: 9 in]
                  }
                  "Array" <- w447
                  n125 = global write "Glob_Ref.vi" "Array_temp"(w447) -> ()
                }
                frame True {
                }
              }
            }
            frame "trigger" {
              n126 = call "fgv_DL950_config.vi"("cmd"=rw."read") -> ("config 2"=w495:T9)  [unwired: 9 in, 1 out]
              n127 = Unbundle By Name(w495) -> ("Trigger on"=w486:bool, "Trig Pos"=w485:dbl, "Trigger Source"=w492:i32, "Trig Mode"=w491:i32, "Trigger Slope"=w487:i32, "Trigger Level"=w490:dbl)
              n128 = case shown="True" w486 {
                tunnel: w494 -> [w498 w509]
                tunnel: w493 -> [w497 w508]
                tunnel: w492 -> [_ w502]
                tunnel: w491 -> [_ w501]
                tunnel: w490 -> [_ w507]
                tunnel: [w497 w504] -> w489
                tunnel: [w498 w503] -> w488
                tunnel: w487 -> [_ w500]
                tunnel: w485 -> [_ w499]
                frame False {
                }
                frame True {
                  n129 = call <instrlib>:"Configure Trigger(Basic).vi"("VISA resource name"=w508, "Trigger Source (1: CH1)"=w502, "Trigger Mode (1: Auto)"=w501, "Trigger Slope (0: Rising)"=w500, "Trigger Level (0)"=w507, "error in (no error)"=w509) -> ("VISA resource name out"=w506:refnum<visa-resource-name>, "error out"=w505:errorcluster)  [unwired: 8 in]
                  n130 = call <instrlib>:"Configure Trigger Position.vi"("VISA resource name"=w506, "Trigger Position (50%)"=w499, "error in (no error)"=w505) -> ("VISA resource name out"=w504:refnum<visa-resource-name>, "error out"=w503:errorcluster)  [unwired: 11 in]
                }
              }
            }
          }
          n131 = Unbundle By Name(w16) -> ("status"=w23:bool)
          n132 = call "fgv_stop_global.vi"("cmd"=init-r-stop."read") -> ("stop"=w20:bool)  [unwired: 10 in]
          n133 = Not(x=w23) -> (.not. x?=w22:bool)
          n134 = Or(x=w22, y=w20) -> (x .or. y?=w21:bool)
        }
      }
      "error out" <- w6
      n135 = call "fgv_Err-Device.vi"("Err Sel"=T3."DL950", "first?"=w4, "cmd"=w5, "error in"=w6) -> ()  [unwired: 8 in]
    }
  }
  n136 = disable-structure shown="Disabled" {
    frame Disabled {
      n137 = call <instrlib>:"VI Tree.vi"() -> ()  [unwired: 12 in]
    }
    frame Enabled {
    }
  }
